vi "3-6.vi"() -> ()   [LabVIEW 2022 SP3]
panel:
  out "文本":string
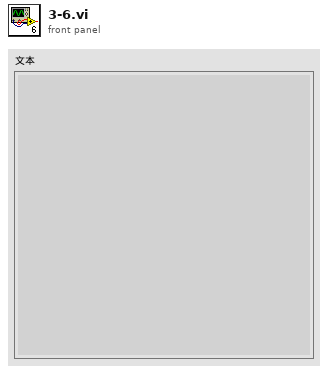
[diagram p1: front panel]
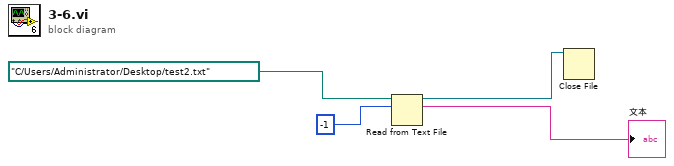
[diagram p0: block diagram]
diagram:
  n1 = Read from Text File(file (use dialog)=path "C:/Users/Administrator/Desktop/test2.txt" ("文件（使用对话框）"), count=-1 ("计数")) -> (refnum out=w1:refnum<file>, text=→"文本":string)  [unwired: 2 in, 2 out]
  n2 = Close File(refnum=w1) -> ()  [unwired: 1 in, 2 out]
